vi "get async cmd.vi"(10 "error in (no error)":errorcluster, 11 "Cmd String in":string) -> (2 "error out":errorcluster, 3 "AsyncCmd":T1)   [LabVIEW 2019, in "DAQ_Engine.lvclass"]
doc: "Developed by Kevin Thompson\nkevin@thompsonengineering.net\n\nCopyright 2018\nThompson Engineering, LLC"
uses:
  DAQ_Engine.lvclass
  DataTypes/AsynCmd_DAQ_Engine--enum.ctl
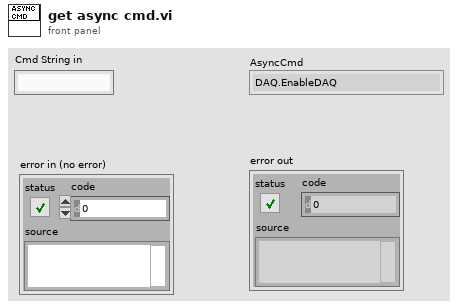
[diagram p1: front panel]
types:
  T1 = typedef "DAQ_Engine.lvclass/AsynCmd_DAQ_Engine--enum.ctl" = enum16{"DAQ.EnableDAQ", "DAQ.ClearDAQError", "DAQ.SetMeasConfig", "DAQ.SetAcqMode", "DAQ.SetErrorReporting"}
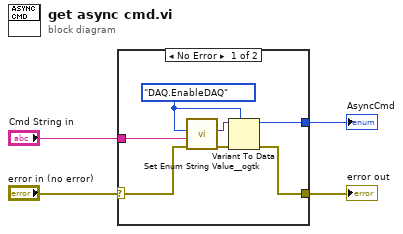
[diagram p0: block diagram]
diagram:
  n1 = case shown="No Error" "error in (no error)" {
    selector: "error in (no error)" -> [w5 w12]
    tunnel: "Cmd String in" -> [w10 _]
    tunnel: [w9 _] -> w3
    tunnel: [w6 w12] -> w2
    frame No Error {
      w8 = AsynCmd_DAQ_Engine--enum."DAQ.EnableDAQ" ("AsyncCmd")
      n2 = call <userlib>:"Set Enum String Value__ogtk.vi"("error in (no error)"=w5, "String Value"=w10, "Default Enum Value"=w8) -> ("error out"=w7:errorcluster, "Enum"=w11:variant)  [unwired: 7 in]
      n3 = Variant To Data(error in=w7, type=w8, Variant=w11) -> (data=w9:T1, error out=w6:errorcluster)
    }
    frame Error {
    }
  }
  "AsyncCmd" <- w3
  "error out" <- w2
